vi "CsLv_GetSystemInfoAll.vi"(0 "Handle":u32) -> (1 "Memory Size":dbl, 2 "Board Type":u32, 3 "Number Of Triggers":u32, 4 "Number Of Channels":u32, 5 "Number Of Boards":u32, 6 "Sample Bits":u32, 7 "Error Code":i32)   [LabVIEW 2022 SP3]
doc: "This VI returns information about the CompuScope system identified by Handle, which is obtained with CsLv_GetSystem.vi. \n\nThe available information is as follows: \n Memory Size (of each CompuScope board in the system)\n Board Type\n Number Of Triggers (number of trigger engines in the system)\n Number Of Channels (in the system)\n Number Of Boards (in the system)\n Sample Bits (vertical resolution for the CompuScope system)\n\nBoard Type is an integer constant used by the CompuScope driver to identify each type of CompuScope board. CsLv_BoardNameToType.vi may be used to determine the Board Type for any CompuScope model.\n\nBoard Type, Number Of Triggers, Number Of Channels, Number Of Boards and Sample Bits are all integer values. Memory Size is a double variable that indicates the amount of on-board CompuScope memory in samples.\n\nIf the call is successful, a 1 is returned in the Error Code indicator. Otherwise, an appropriate error code is returned. A descriptive error string may be obtained by using CsLv_GetErrorString.vi."
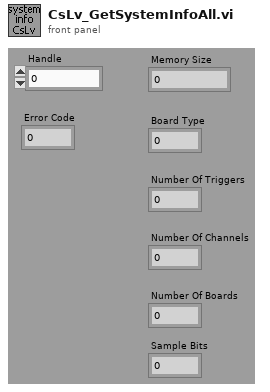
[diagram p1: front panel]
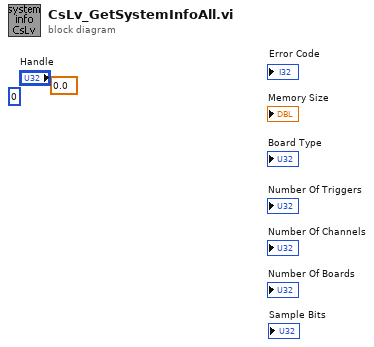
[diagram p0: block diagram]
diagram:
  (unwired) u32 0
  (unwired) 0.0
